vi "Read Runtime Specific Configuration.vi"(8 "error in (no error)":errorcluster, 11 "E2E Tag Exchange configuration in":refnum<class "E2E Tag Exchange configuration.lvclass">) -> (0 "error out":errorcluster, 2 "Runtime Specific Configuration":variant, 3 "E2E Tag Exchange configuration out":refnum<class "E2E Tag Exchange configuration.lvclass">)   [LabVIEW 2015, in "E2E Tag Exchange configuration.lvclass"]
uses:
  E2E Tag Exchange configuration.lvclass
  E2E Tag Exchange configuration.lvclass/E2E Tag Exchange configuration.ctl
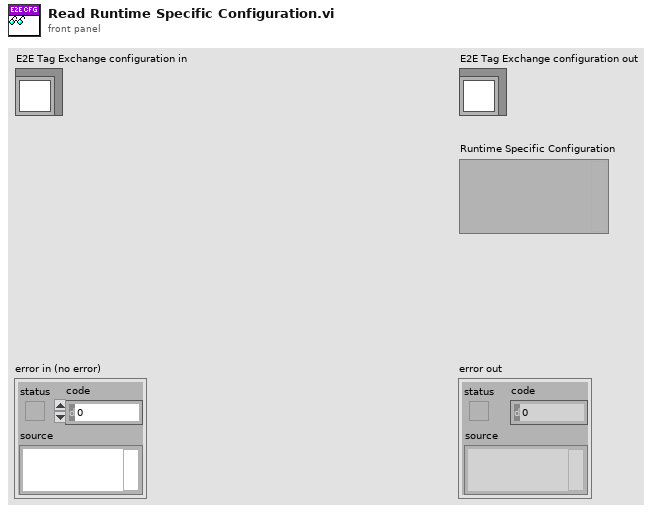
[diagram p1: front panel]
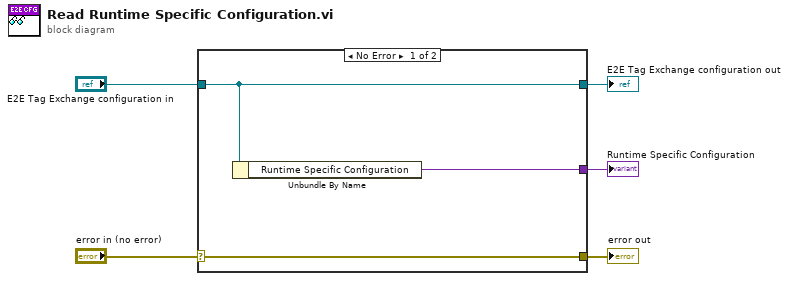
[diagram p0: block diagram]
diagram:
  n1 = case shown="No Error" "error in (no error)" {
    selector: "error in (no error)" -> [w8 w9]
    tunnel: [w8 w9] -> w4
    tunnel: [w7 w10] -> w2
    tunnel: "E2E Tag Exchange configuration in" -> [w7 w10]
    tunnel: [w6 _] -> w1
    frame No Error {
      n2 = Unbundle By Name(w7) -> ("Runtime Specific Configuration"=w6:variant)
    }
    frame Error {
    }
  }
  "error out" <- w4
  "E2E Tag Exchange configuration out" <- w2
  "Runtime Specific Configuration" <- w1
